vi "Cancel Send.vi"(8 "error in (no error)":errorcluster, 11 "Repeat Message Control in":refnum<class "Repeat Message Control.lvclass">) -> (0 "error out":errorcluster, 3 "Repeat Message Control out":refnum<class "Repeat Message Control.lvclass">)   [LabVIEW 2020, in "Volatus.lvlib" / "Repeat Message Control.lvclass"]
uses:
  Repeat Message Control.lvclass
  Repeat Message Control.lvclass/Repeat Message Control.ctl
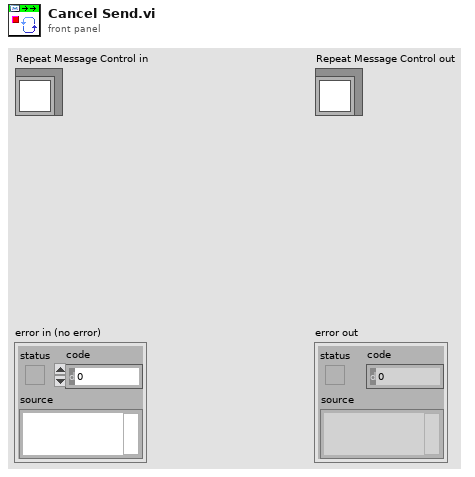
[diagram p1: front panel]
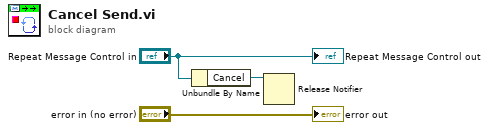
[diagram p0: block diagram]
diagram:
  n1 = Unbundle By Name("Repeat Message Control in") -> ("Cancel"=w1:refnum<notifier>)
  n2 = Release Notifier(notifier=w1) -> ()  [unwired: 2 in, 3 out]
  "error out" <- "error in (no error)"
  "Repeat Message Control out" <- "Repeat Message Control in"
